vi "ReceiveUDPEth.vi"(3 "Cnt in":u32, 4 "Boot_proc":bool=TRUE, 5 "queue out":refnum<queue>, 6 "connection ID":refnum<k16>) -> (0 "unsigned byte array":u8[](array[numeric]), 1 "Cnt out":u32, 2 "sts_E_T":bool)   [LabVIEW 2017]
panel:
  out "error out 2":errorcluster
  out "counter":u32
  out "error out":errorcluster
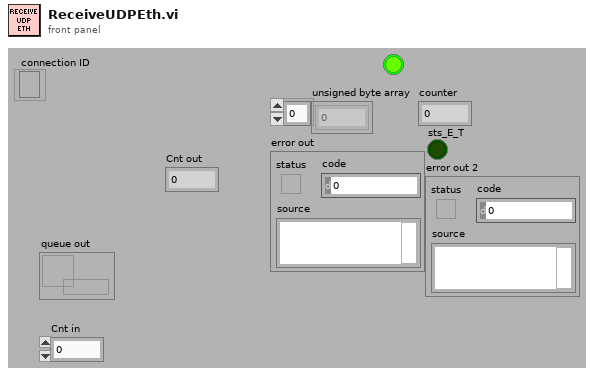
[diagram p1: front panel]
types:
  T1 = cluster{"ID":u32, "MSGTYPE":u8, "LEN":u8, "aDATA":u8[]}
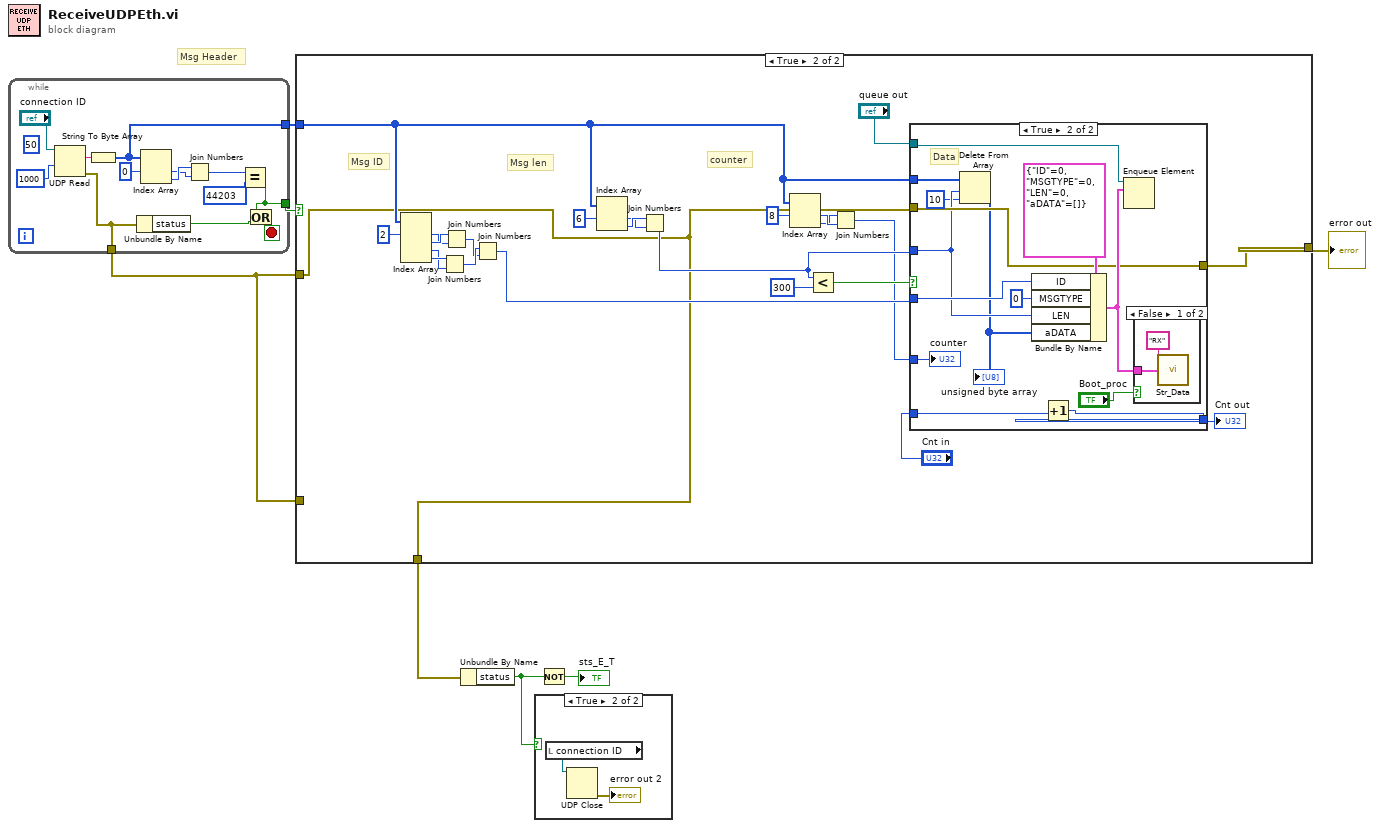
[diagram p0: block diagram]
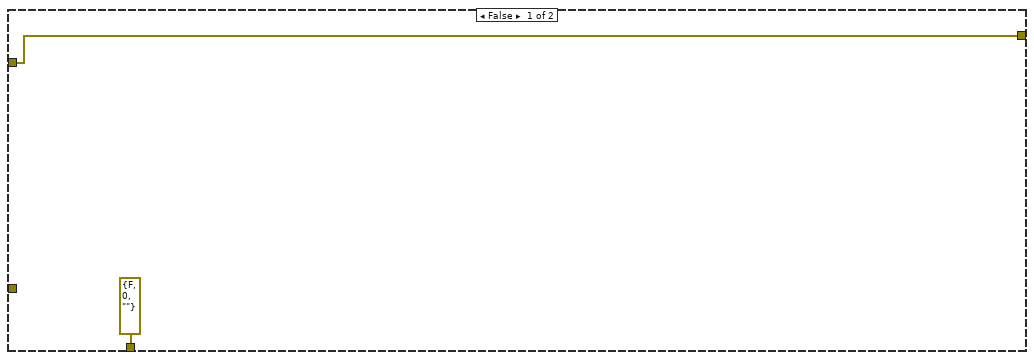
[diagram p3: hidden frame]
diagram:
  # "Msg Header"
  n1 = while {
    tunnel: [w19] -> w6
    tunnel: [w14] -> w4
    tunnel: [w10] -> w3
    stop <- w20 stop-if-true
    (unwired) 50
    n2 = UDP Read(connection ID="connection ID", timeout ms (25000)=1000) -> (data out=w13:string, error out=w14:errorcluster)  [unwired: 2 in, 3 out]
    n3 = String To Byte Array(string=w13) -> (unsigned byte array=w10:u8[])
    n4 = Unbundle By Name(w14) -> ("status"=w15:bool)
    n5 = Index Array(array=w10, index #1=0 ("index")) -> (element #1=w8:u8, element #2=w9:u8)  [unwired: 1 in]
    n6 = Join Numbers(hi=w9, lo=w8) -> ((hi.lo)=w11:u16)
    n7 = Equal?(x=w11, y=u16 44203) -> (x = y?=w19:bool)
    n8 = Or(x=w19, y=w15) -> (x .or. y?=w20:bool)
  }
  n9 = case shown="True" w6 {
    tunnel: w4 -> [w22 w24]
    tunnel: [w22 w33] -> w7
    tunnel: [errorcluster {"status"=FALSE, "code"=0, "source"=""} ("error out") w24] -> w5
    tunnel: w4 -> [_ _]
    tunnel: w3 -> [_ w25]
    frame False {
    }
    frame True {
      # "counter"
      # "Msg ID"
      # "Msg len"
      n10 = Index Array(array=w25, index #1=2 ("index")) -> (element #1=w38:u8, element #2=w39:u8, element #3=w40:u8, element #4=w41:u8)  [unwired: 3 in]
      n11 = Join Numbers(hi=w41, lo=w40) -> ((hi.lo)=w43:u16)
      n12 = Join Numbers(hi=w39, lo=w38) -> ((hi.lo)=w42:u16)
      n13 = Join Numbers(hi=w43, lo=w42) -> ((hi.lo)=w28:u32)
      n14 = Index Array(array=w25, index #1=6 ("index")) -> (element #1=w35:u8, element #2=w36:u8)  [unwired: 1 in]
      n15 = Join Numbers(hi=w36, lo=w35) -> ((hi.lo)=w27:u16)
      n16 = Index Array(array=w25, index #1=8 ("index")) -> (element #1=w30:u8, element #2=w29:u8)  [unwired: 1 in]
      n17 = Less?(x=w27, y=300) -> (x < y?=w45:bool)
      n18 = Join Numbers(hi=w29, lo=w30) -> ((hi.lo)=w23:u16)
      n19 = case shown="True" w45 {
        tunnel: "queue out" -> [_ w61]
        tunnel: "Cnt in" -> [w48 w57]
        tunnel: [w48 w56] -> w46
        tunnel: w27 -> [_ w52]
        tunnel: w28 -> [_ w58]
        tunnel: w24 -> [w47 w54]
        tunnel: [w47 w54] -> w33
        tunnel: w23 -> [_ w55]
        tunnel: w25 -> [_ w53]
        frame False {
        }
        frame True {
          # "Data"
          n20 = Delete From Array(array=w53, length=w52, index=10) -> (deleted portion=w50:u8[])  [unwired: 1 out]
          "unsigned byte array" <- w50
          n21 = Bundle By Name(cluster=T1 {"ID"=0, "MSGTYPE"=0, "LEN"=0, "aDATA"=[]} ("Msg"), "ID"=w58, "MSGTYPE"=u8 0, "LEN"=w52, "aDATA"=w50) -> (w60:T1)
          n22 = Increment(x=w57) -> (x+1=w56:u32)
          n23 = Enqueue Element(queue=w61, element=w60) -> ()  [unwired: 1 in, 4 out]
          n24 = case shown="False" "Boot_proc" {
            tunnel: w60 -> [w63 _]
            frame False {
              n25 = call "Str_Data.vi"("Msg"=w63, "string"="RX") -> ()  [unwired: 1 in, 1 out]
            }
            frame True {
            }
          }
          "counter" <- w55
        }
      }
      "Cnt out" <- w46
    }
  }
  "error out" <- w7
  n26 = Unbundle By Name(w5) -> ("status"=w2:bool)
  n27 = case shown="True" w2 {
    frame False {
    }
    frame True {
      n28 = local read "connection ID"() -> (w66:refnum<k16>)
      n29 = UDP Close(connection ID=w66) -> (error out=→"error out 2":errorcluster)  [unwired: 1 in, 1 out]
    }
  }
  n30 = Not(x=w2) -> (.not. x?=→"sts_E_T":bool)
